vi "read pixels.vi"(0 "fpga interface in":refnum<k20>, 1 "image queue in":refnum<queue>, 5 "display channel number":i32, 7 "serial channel display parameters":T4[](array[typedef]) {"RAW parameters"."bayer parameters"."blue gain" format="%_4g"; "RAW parameters"."bayer parameters"."green gain" format="%_4g"; "RAW parameters"."bayer parameters"."red gain" format="%_4g"; "RAW parameters"."bayer parameters"."algorithm" items=["Bilinear", "VNG"]; "RAW parameters"."bayer parameters"."pattern" items=["GB", "GR", "BG", "RG"]}, 9 "image metadata":T2, 11 "error in (no error)":errorcluster) -> (4 "fpga interface out":refnum<k20>, 6 "display image":T1, 15 "error out":errorcluster)   [LabVIEW 2025, in "Automotive Vision.lvclass"]
uses:
  Automotive Vision.lvclass
  Automotive Vision.lvclass/Automotive Vision.ctl
  Program Files/NI/LVAddons/flexrioii/1/ProjectTemplates/Source/FlexRIO/NI148X/Getting Started/Host/Common/GettingStarted_Common_148X_Host.lvlib
  <instrlib>/FlexRIO/CSI-2/v2/Common/Types/LLP Data Type.ctl
  <instrlib>/FlexRIO/CSI-2/v2/Common/NI CSI-2 API Common v2.lvlib
  image.ctl
  <vilib>/vision/Image Controls.llb/IMAQ Image.ctl
  Program Files/NI/LVAddons/flexrioii/1/ProjectTemplates/Source/FlexRIO/NI148X/Getting Started/Host/Common/Types/RAW Interpretation for Display.ctl
  Program Files/NI/LVAddons/flexrioii/1/ProjectTemplates/Source/FlexRIO/NI148X/Getting Started/Host/Common/Types/Serial Channel Display Parameters.ctl
  Program Files/NI/LVAddons/flexrioii/1/ProjectTemplates/Source/FlexRIO/NI148X/Getting Started/FPGA/Common/Types/Image Metadata.ctl
  Program Files/NI/LVAddons/flexrioii/1/ProjectTemplates/Source/FlexRIO/NI148X/Getting Started/FPGA/Common/GettingStarted_Common_148X_FPGA.lvlib
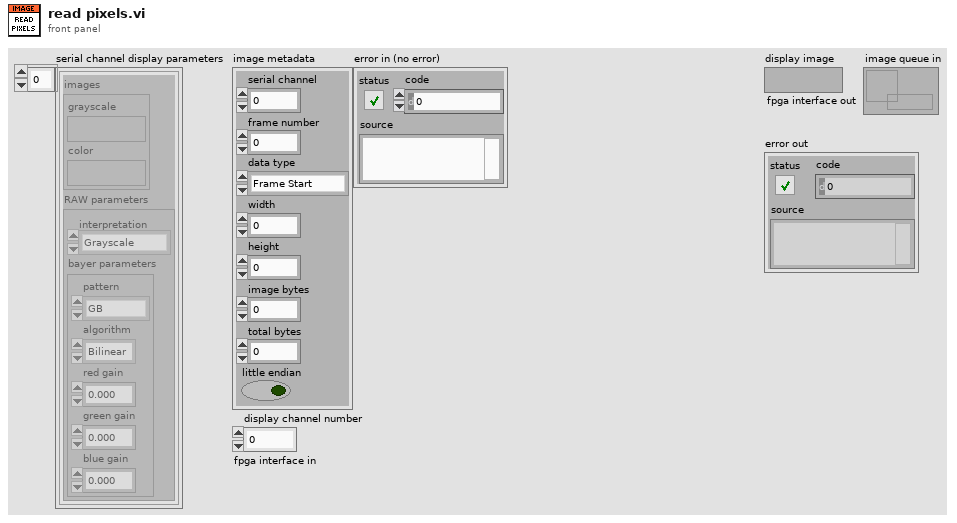
[diagram p1: front panel]
types:
  T1 = typedef "IMAQ Image.ctl" = refnum<image>
  T2 = typedef "GettingStarted_Common_148X_FPGA.lvlib/Image Metadata.ctl" = cluster{"serial channel":fxp<+,3,3>, "frame number":u16, "data type":T3, "width":u16, "height":u16, "image bytes":u32, "total bytes":u32, "little endian":bool}
  T3 = typedef "NI CSI-2 API Common v2.lvlib/LLP Data Type.ctl" = enum8{"Frame Start", "Frame End", "Line Start", "Line End", "End of Transmission", "Reserved 0", "Reserved 1", "Reserved 2", "Generic Short Packet 1", "Generic Short Packet 2", "Generic Short Packet 3", "Generic Short Packet 4", "Generic Short Packet 5", "Generic Short Packet 6", "Generic Short Packet 7", "Generic Short Packet 8", "Null", "Blanking Data", "Embedded 8-bit non Image Data", "Generic Long Packet 1", "Generic Long Packet 2", "Generic Long Packet 3", "Generic Long Packet 4", "Reserved 3", "YUV420 8-bit", "YUV420 10-bit", "Legacy YUV420 8-bit", "Reserved 4", "YUV420 8-bit Chroma Shifted", "YUV420 10-bit Chroma Shifted", "YUV422 8-bit", "YUV422 10-bit", "RGB444", "RGB555", "RGB565", "RGB666", "RGB888", "Reserved 5", "Reserved 6", "RAW 24", "RAW 6", "RAW 7", "RAW 8", "RAW 10", "RAW 12", "RAW 14", "RAW 16", "RAW 20", "User Defined 8-bit Data 1", "User Defined 8-bit Data 2", "User Defined 8-bit Data 3", "User Defined 8-bit Data 4", "User Defined 8-bit Data 5", "User Defined 8-bit Data 6", "User Defined 8-bit Data 7", "User Defined 8-bit Data 8", "USL Command", "Reserved 7", "Reserved 8", "Reserved 9", "Reserved 10", "Reserved 11", "Reserved 12", "LRTE EPD Spacer"}
  T4 = typedef "GettingStarted_Common_148X_Host.lvlib/Serial Channel Display Parameters.ctl" = cluster{"images":cluster{"grayscale":T1, "color":T1}, "RAW parameters":cluster{"interpretation":T5, "bayer parameters":cluster{"pattern":i32, "algorithm":i32, "red gain":dbl, "green gain":dbl, "blue gain":dbl}}}
  T5 = typedef "GettingStarted_Common_148X_Host.lvlib/RAW Interpretation for Display.ctl" = enum16{"Grayscale", "Bayer", "RGB", "YUV422", "YUV420", "Legacy YUV420"}
  T6 = typedef "Automotive Vision.lvclass/image.ctl" = cluster{"Frame ID":u32, "Data":u8[]}
  T7 = cluster{"pattern":i32, "algorithm":i32, "red gain":dbl, "green gain":dbl, "blue gain":dbl}
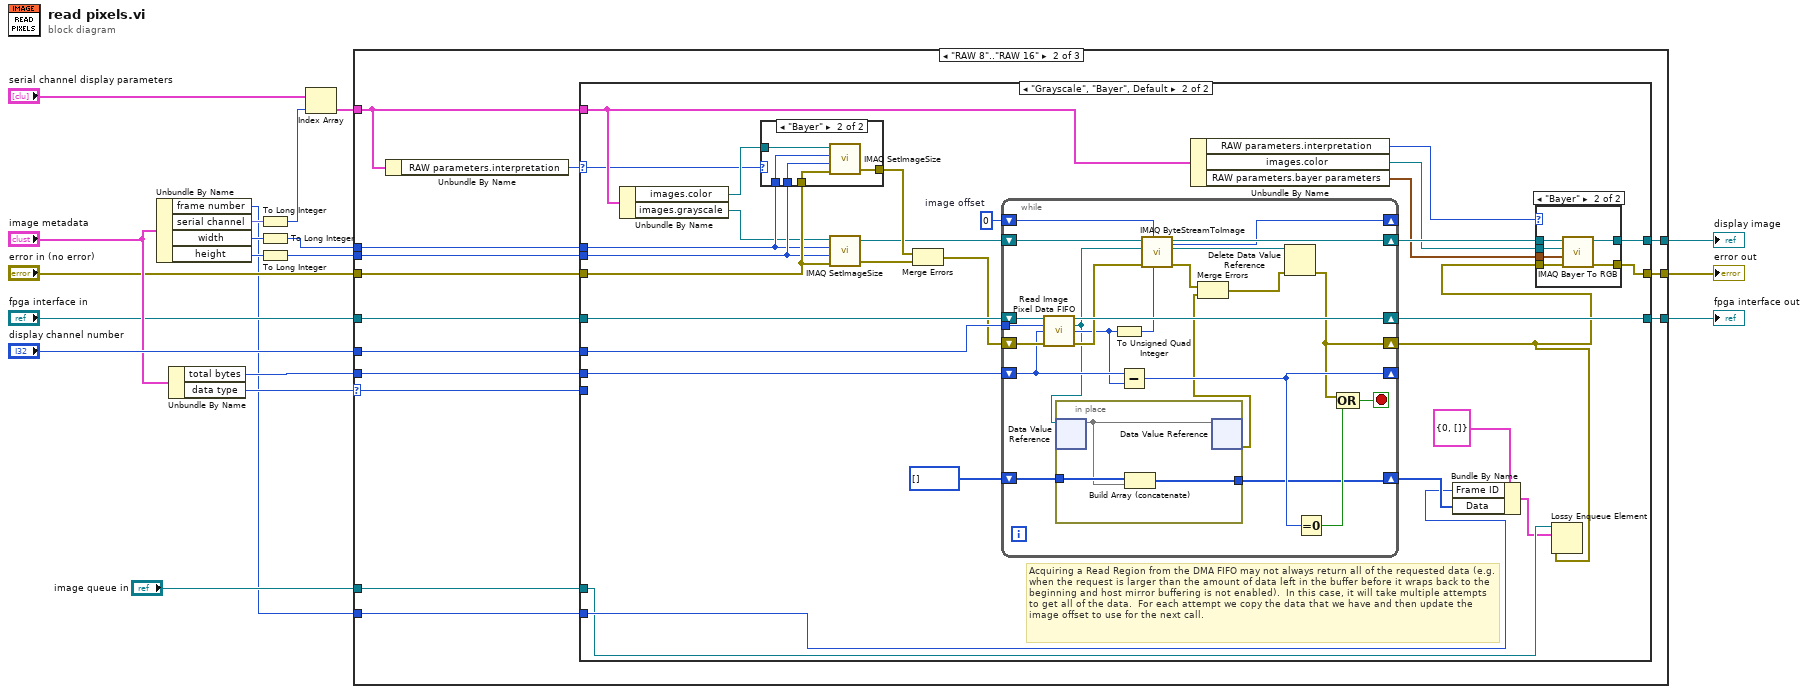
[diagram p0: block diagram]
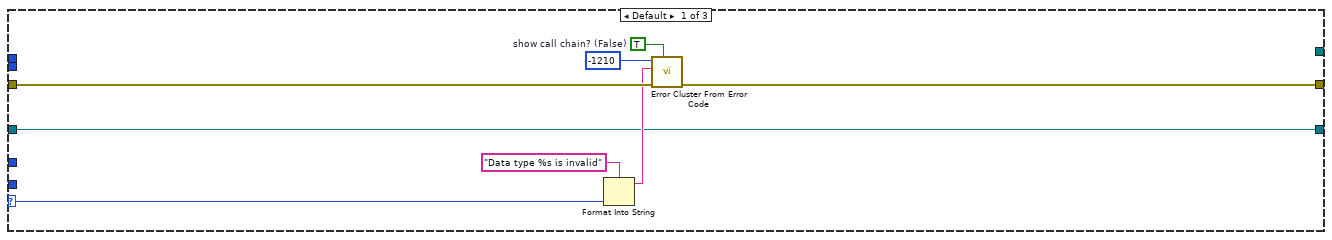
[diagram p2: hidden frame]
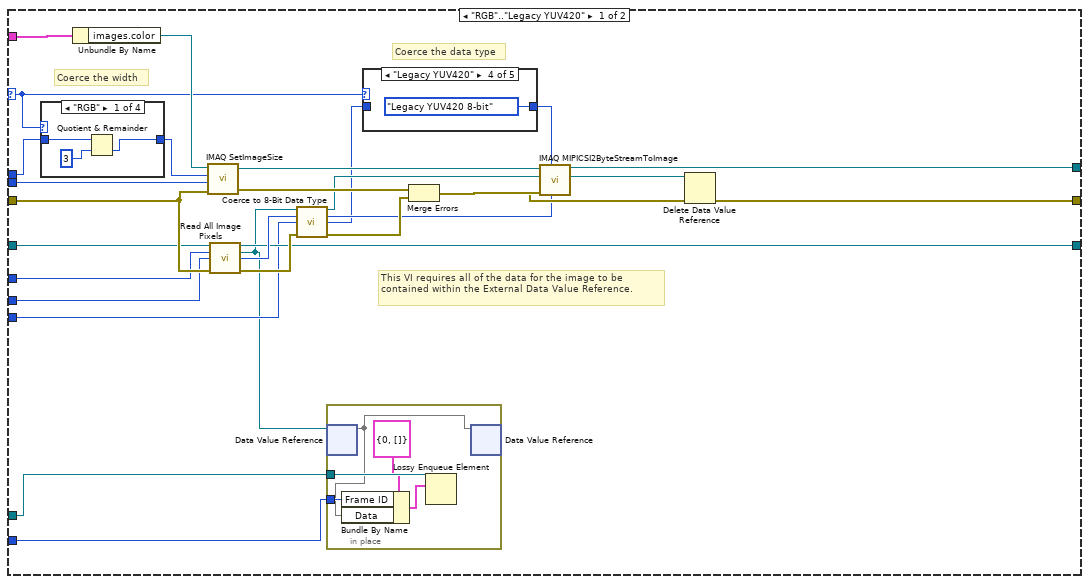
[diagram p3: hidden frame]
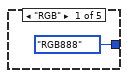
[diagram p4: hidden frame]
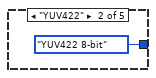
[diagram p5: hidden frame]
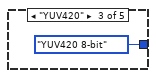
[diagram p6: hidden frame]
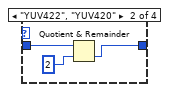
[diagram p8: hidden frame]
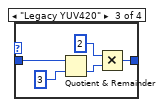
[diagram p9: hidden frame]
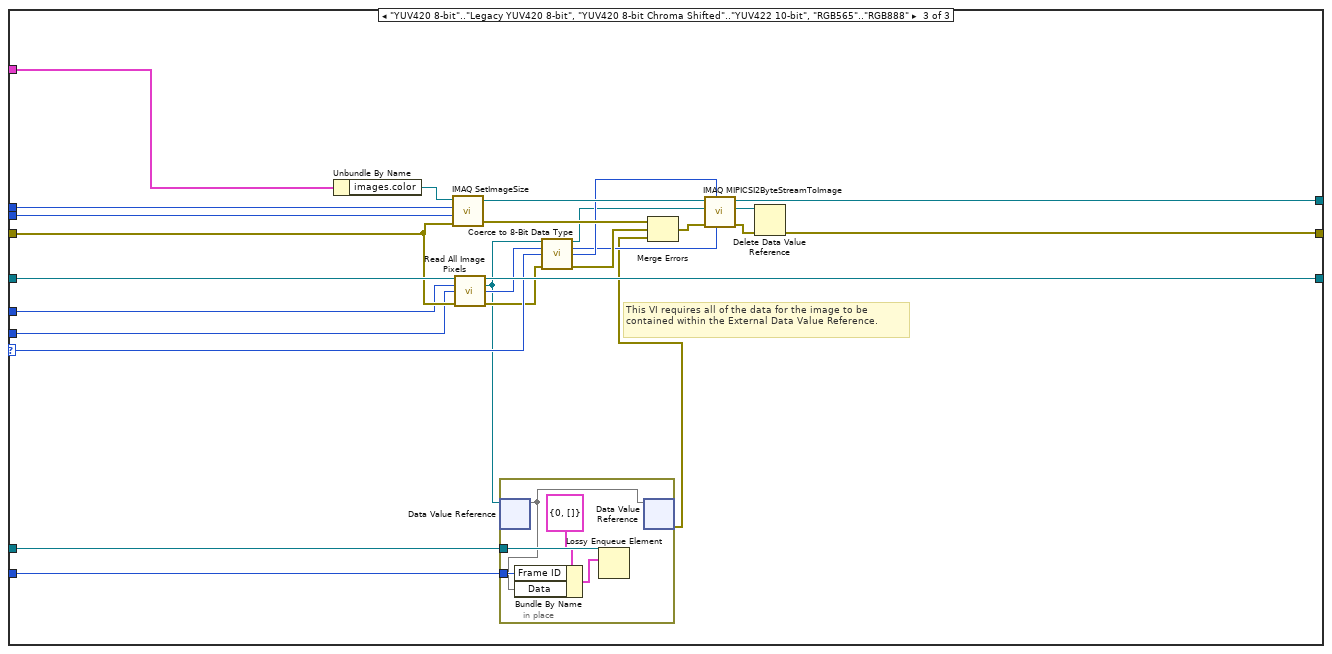
[diagram p13: hidden frame]
diagram:
  n1 = Unbundle By Name("image metadata") -> ("frame number"=w1:u16, "serial channel"=w15:fxp<+,3,3>, "width"=w11:u16, "height"=w12:u16)
  n2 = Unbundle By Name("image metadata") -> ("total bytes"=w18:u32, "data type"=w3:T3)
  n3 = To Long Integer(number=w15) -> (32bit integer=w13:i32)
  n4 = To Long Integer(number=w11) -> (32bit integer=w8:i32)
  n5 = To Long Integer(number=w12) -> (32bit integer=w9:i32)
  n6 = Index Array(array="serial channel display parameters", index=w13) -> (element=w5:T4)
  n7 = case shown="\"RAW 8\"..\"RAW 16\"" w3 {
    selector: w3 -> [w21 w30 w170]
    tunnel: w18 -> [_ w41 w178]
    tunnel: [w20 w40 w180] -> w17
    tunnel: "display channel number" -> [_ w39 w177]
    tunnel: "error in (no error)" -> [w25 w38 w181]
    tunnel: w9 -> [_ w37 w188]
    tunnel: w8 -> [_ w36 w187]
    tunnel: [_ w35 w176] -> w7
    tunnel: [w24 w34 w173] -> w6
    tunnel: w5 -> [_ w32 w185]
    tunnel: "fpga interface in" -> [w20 w33 w184]
    tunnel: "image queue in" -> [_ w29 w163]
    tunnel: w1 -> [_ w28 w162]
    frame Default {
      w26 = TRUE  # show call chain? (False)
      n8 = Format Into String(format string="Data type %s is invalid" ("error message (\"\")"), w21) -> (resulting string=w22:string)  [unwired: 2 in, 1 out]
      n9 = call <vilib>:"Error Cluster From Error Code.vi"("show call chain? (False)"=w26, "error in (no error)"=w25, "error message (\"\")"=w22, "error code (0)"=-1210) -> ("error out"=w24:errorcluster)  [unwired: 5 in]
    }
    frame "RAW 8".."RAW 16" {
      n10 = Unbundle By Name(w32) -> ("RAW parameters.interpretation"=w31:T5)
      n11 = case shown="\"Grayscale\", \"Bayer\", Default" w31 {
        selector: w31 -> [w47 w100]
        tunnel: w41 -> [w54 w121]
        tunnel: [w58 w119] -> w40
        tunnel: w39 -> [w53 w118]
        tunnel: w38 -> [w59 w117]
        tunnel: w37 -> [w50 w115]
        tunnel: w36 -> [w49 w114]
        tunnel: [w56 w111] -> w35
        tunnel: [w57 w110] -> w34
        tunnel: w32 -> [w52 w105]
        tunnel: w33 -> [w55 w104]
        tunnel: w30 -> [w51 _]
        tunnel: w29 -> [w43 w95]
        tunnel: w28 -> [w42 w96]
        frame "RGB".."Legacy YUV420" {
          # "Coerce the data type"
          # "Coerce the width"
          # "This VI requires all of the data for the image to be contained within the External Data Value Reference."
          n12 = case shown="\"RGB\"" w47 {
            tunnel: w49 -> [w82 w85 w91 w92]
            tunnel: [w81 w84 w88 w92] -> w48
            frame "RGB" {
              n13 = Quotient & Remainder(x=w82, y=3) -> (floor(x/y)=w81:i32)  [unwired: 1 out]
            }
            frame "YUV422", "YUV420" {
              n14 = Quotient & Remainder(x=w85, y=2) -> (floor(x/y)=w84:i32)  [unwired: 1 out]
            }
            frame "Legacy YUV420" {
              n15 = Quotient & Remainder(x=w91, y=3) -> (floor(x/y)=w89:i32)  [unwired: 1 out]
              n16 = Multiply(x=2, y=w89) -> (x*y=w88:i32)
            }
            frame Default {
            }
          }
          n17 = Unbundle By Name(w52) -> ("images.color"=w70:T1)
          n18 = call "IMAQ SetImageSize"("error in (no error)"=w59, "Y Resolution"=w50, "X Resolution"=w48, "Image"=w70) -> ("error out"=w68:errorcluster, "Image Out"=w69:T1)  [unwired: 1 in]
          n19 = call "Read All Image Pixels.vi"("fpga inteface in"=w55, "display channel number"=w53, "image bytes"=w54, "error in (no error)"=w59) -> ("fpga interface out"=w58:refnum<k20>, "image pixel data region"=w44:refnum<data-value>, "elements in region"=w63:u32, "error out"=w64:errorcluster)  [unwired: 8 in]
          n20 = call "Coerce to 8-Bit Data Type.vi"("image pixel data region in"=w44, "image bytes in"=w63, "data type in"=w51, "error in (no error)"=w64) -> ("image pixel data region out"=w60:refnum<data-value>, "image bytes out"=w61:u32, "data type out"=w45:T3, "error out"=w62:errorcluster)  [unwired: 8 in]
          n21 = in-place {
            in-place-border: w43 -> [w75]
            in-place-border: w42 -> [w72]
            n22 = in-place-dvr #1(w44) -> (w71:u8[])  [unwired: 1 out]
            n23 = Bundle By Name(cluster=T6 {"Frame ID"=0, "Data"=[]} ("Image"), "Frame ID"=w72, "Data"=w71) -> (w73:T6)
            n24 = Lossy Enqueue Element(queue=w75, element=w73) -> ()  [unwired: 1 in, 4 out]
            n25 = in-place-dvr #1(w71) -> ()  [unwired: 2 out]
          }
          n26 = case shown="\"Legacy YUV420\"" w47 {
            tunnel: w45 -> [_ _ _ _ w80]
            tunnel: [LLP_Data_Type."RGB888" ("data type") LLP_Data_Type."YUV422 8-bit" ("data type") LLP_Data_Type."YUV420 8-bit" ("data type") LLP_Data_Type."Legacy YUV420 8-bit" ("data type") w80] -> w46
            frame "RGB" {
            }
            frame "YUV422" {
            }
            frame "YUV420" {
            }
            frame "Legacy YUV420" {
            }
            frame Default {
            }
          }
          n27 = Merge Errors(w68, w62) -> (w67:errorcluster)
          n28 = call "IMAQ MIPICSI2ByteStreamToImage"("Bytes to Copy"=w61, "Format"=w46, "error in (no error)"=w67, "Byte Stream In"=w60, "Image In"=w69) -> ("error out"=w66:errorcluster, "Byte Stream Out"=w65:refnum<data-value>, "Image Out"=w56:T1)  [unwired: 3 in, 1 out]
          n29 = Delete Data Value Reference(data value reference=w65, error in=w66) -> (error out=w57:errorcluster)  [unwired: 1 out]
        }
        frame "Grayscale", "Bayer", Default {
          w101 = u32 0  # image offset
          # "Acquiring a Read Region from the DMA FIFO may not always return all of the requested data (e.g. when the request is larger than the amount of data left in the buffer before it wraps back to the beginning and host mirror buffering is not enabled).  In this case, it will take multiple attempts to get all of the data.  For each attempt we copy the data that we have and then update the image offset to use for the next call."
          n30 = Unbundle By Name(w105) -> ("images.color"=w113:T1, "images.grayscale"=w109:T1)
          n31 = case shown="\"Bayer\"" w100 {
            tunnel: w117 -> [w122 w127]
            tunnel: [w122 w126] -> w116
            tunnel: w113 -> [_ w125]
            tunnel: w115 -> [_ w124]
            tunnel: w114 -> [_ w123]
            frame "Grayscale", Default {
            }
            frame "Bayer" {
              n32 = call "IMAQ SetImageSize"("error in (no error)"=w127, "Y Resolution"=w124, "X Resolution"=w123, "Image"=w125) -> ("error out"=w126:errorcluster)  [unwired: 1 in, 1 out]
            }
          }
          n33 = call "IMAQ SetImageSize"("error in (no error)"=w117, "Y Resolution"=w115, "X Resolution"=w114, "Image"=w109) -> ("error out"=w120:errorcluster, "Image Out"=w103:T1)  [unwired: 1 in]
          n34 = Merge Errors(w116, w120) -> (w102:errorcluster)
          n35 = while {
            tunnel: w118 -> [w148]
            shift-right: [w149] -> w119
            shift-left: w104 -> [w150]
            shift-right: [w136] -> w93
            shift-left: w102 -> [w147]
            shift-right: [w145] -> w112
            shift-left: w103 -> [w146]
            shift-right: [w139] -> _
            shift-left: w121 -> [w141]
            shift-right: [w135] -> _
            shift-left: w101 -> [w134]
            shift-right: [w128] -> w97
            shift-left: u8[] [] ("Data") -> [w129]
            stop <- w137 stop-if-true
            n36 = call "Read Image Pixel Data FIFO.vi"("fpga inteface in"=w150, "display channel number"=w148, "number of elements"=w141, "error in (no error)"=w147) -> ("fpga interface out"=w149:refnum<k20>, "image pixel data region"=w133:refnum<data-value>, "elements in region"=w140:u32, "error out"=w144:errorcluster)  [unwired: 7 in, 1 out]
            n37 = in-place {
              in-place-border: w129 -> [w153]
              in-place-border: [w152] -> w128
              n38 = in-place-dvr #2(w133) -> (w151:u8[])  [unwired: 1 out]
              n39 = Build Array (concatenate)(w153, w151) -> (w152:u8[])
              n40 = in-place-dvr #2(w151) -> (w131:errorcluster)  [unwired: 1 out]
            }
            n41 = To Unsigned Quad Integer(1:w140) -> (0:w143:u64)
            n42 = Subtract(x=w141, y=w140) -> (x-y=w139:u32)
            n43 = call "IMAQ ByteStreamToImage"("Bytes to Copy"=w143, "Image Byte Offset In"=w134, "error in (no error)"=w144, "Byte Stream In"=w133, "Image In"=w146) -> ("error out"=w132:errorcluster, "Byte Stream Out"=w142:refnum<data-value>, "Image Out"=w145:T1, "Image Byte Offset Out"=w135:u32)  [unwired: 2 in, 1 out]
            n44 = Merge Errors(w132, w131) -> (w130:errorcluster)
            n45 = Delete Data Value Reference(data value reference=w142, error in=w130) -> (error out=w136:errorcluster)  [unwired: 1 out]
            n46 = Equal To 0?(x=w139) -> (x = 0?=w138:bool)
            n47 = Compound Arithmetic op=OR(w136, w138) -> (w137:bool)
          }
          n48 = Unbundle By Name(w105) -> ("RAW parameters.interpretation"=w106:T5, "images.color"=w107:T1, "RAW parameters.bayer parameters"=w108:T7)
          n49 = Bundle By Name(cluster=T6 {"Frame ID"=0, "Data"=[]} ("Image"), "Frame ID"=w96, "Data"=w97) -> (w94:T6)
          n50 = case shown="\"Bayer\"" w106 {
            tunnel: w112 -> [w154 w161]
            tunnel: [w154 w160] -> w111
            tunnel: w93 -> [w155 w159]
            tunnel: [w155 w158] -> w110
            tunnel: w107 -> [_ w157]
            tunnel: w108 -> [_ w156]
            frame "Grayscale", Default {
            }
            frame "Bayer" {
              n51 = call "IMAQ Bayer To RGB"("error in (no error)"=w159, "Bayer Parameters"=w156, "Image Dst"=w157, "Image Src"=w161) -> ("error out"=w158:errorcluster, "Image Dst Out"=w160:T1)  [unwired: 6 in]
            }
          }
          n52 = Lossy Enqueue Element(queue=w95, element=w94, error in (no error)=w93) -> ()  [unwired: 4 out]
        }
      }
    }
    frame "YUV420 8-bit".."Legacy YUV420 8-bit", "YUV420 8-bit Chroma Shifted".."YUV422 10-bit", "RGB565".."RGB888" {
      # "This VI requires all of the data for the image to be contained within the External Data Value Reference."
      n53 = Unbundle By Name(w185) -> ("images.color"=w186:T1)
      n54 = call "IMAQ SetImageSize"("error in (no error)"=w181, "Y Resolution"=w188, "X Resolution"=w187, "Image"=w186) -> ("error out"=w182:errorcluster, "Image Out"=w183:T1)  [unwired: 1 in]
      n55 = call "Read All Image Pixels.vi"("fpga inteface in"=w184, "display channel number"=w177, "image bytes"=w178, "error in (no error)"=w181) -> ("fpga interface out"=w180:refnum<k20>, "image pixel data region"=w165:refnum<data-value>, "elements in region"=w172:u32, "error out"=w166:errorcluster)  [unwired: 8 in]
      n56 = in-place {
        in-place-border: w163 -> [w193]
        in-place-border: w162 -> [w190]
        n57 = in-place-dvr #3(w165) -> (w189:u8[])  [unwired: 1 out]
        n58 = Bundle By Name(cluster=T6 {"Frame ID"=0, "Data"=[]} ("Image"), "Frame ID"=w190, "Data"=w189) -> (w191:T6)
        n59 = Lossy Enqueue Element(queue=w193, element=w191) -> ()  [unwired: 1 in, 4 out]
        n60 = in-place-dvr #3(w189) -> (w164:errorcluster)  [unwired: 1 out]
      }
      n61 = call "Coerce to 8-Bit Data Type.vi"("image pixel data region in"=w165, "image bytes in"=w172, "data type in"=w170, "error in (no error)"=w166) -> ("image pixel data region out"=w167:refnum<data-value>, "image bytes out"=w168:u32, "data type out"=w169:T3, "error out"=w171:errorcluster)  [unwired: 8 in]
      n62 = Merge Errors(w182, w171, w164) -> (w179:errorcluster)
      n63 = call "IMAQ MIPICSI2ByteStreamToImage"("Bytes to Copy"=w168, "Format"=w169, "error in (no error)"=w179, "Byte Stream In"=w167, "Image In"=w183) -> ("error out"=w175:errorcluster, "Byte Stream Out"=w174:refnum<data-value>, "Image Out"=w176:T1)  [unwired: 3 in, 1 out]
      n64 = Delete Data Value Reference(data value reference=w174, error in=w175) -> (error out=w173:errorcluster)  [unwired: 1 out]
    }
  }
  "display image" <- w7
  "fpga interface out" <- w17
  "error out" <- w6
